vi "Build Blocks Tree.vi"(8 "error in (no error)":errorcluster, 10 "Blocks Map":map{string, T1}(c390), 11 "Blocks Tree":refnum<vi>) -> (0 "error out":errorcluster)   [LabVIEW 2022 SP3, in "FlexBlocks Support.lvlib"]
uses:
  FlexBlocks Support.lvlib
  Worker Info.ctl
  <vilib>/picture/picture.llb/imagedata.ctl
  Worker Variant.ctl
  <vilib>/Utility/miscctls.llb/LVMapReplaceAction.ctl
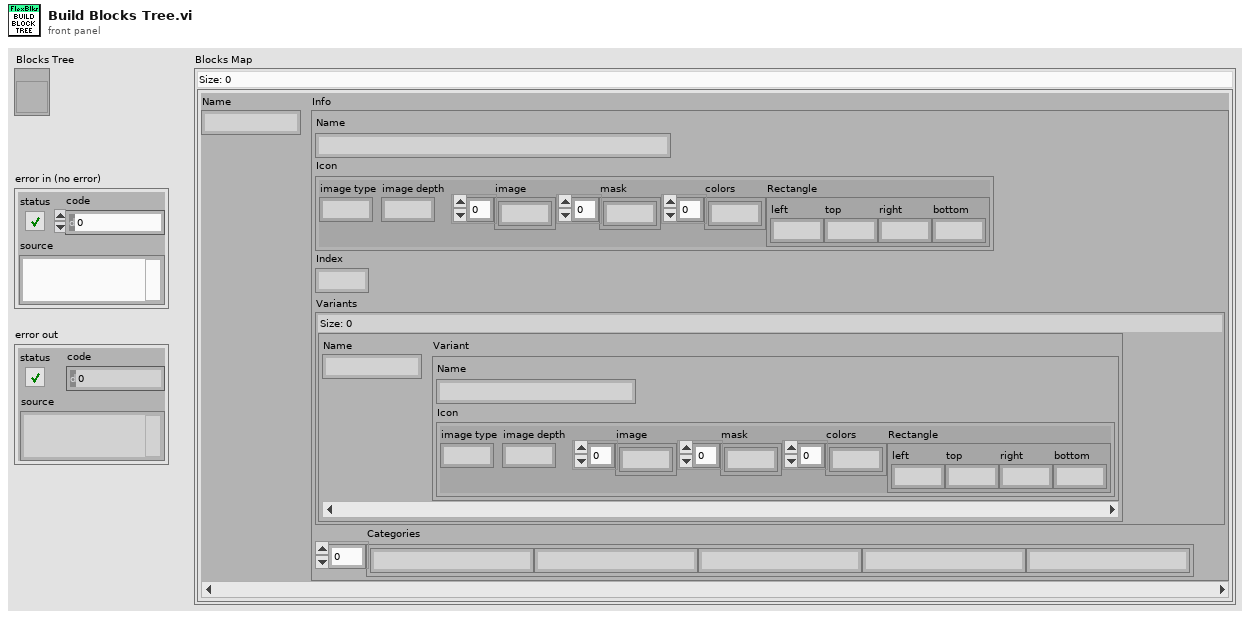
[diagram p1: front panel]
types:
  T1 = typedef "FlexBlocks Support.lvlib/Worker Info.ctl" = cluster{"Name":string, "Icon":T2, "Index":i32, "Variants":map{string, T3}, "Categories":string[]}
  T2 = typedef "imagedata.ctl" = cluster{"image type":i32, "image depth":i32, "image":u8[], "mask":u8[], "colors":u32[], "Rectangle":cluster{"left":i16, "top":i16, "right":i16, "bottom":i16}}
  T3 = typedef "FlexBlocks Support.lvlib/Worker Variant.ctl" = cluster{"Name":string, "Icon":T2}
  T4 = typedef "LVMapReplaceAction.ctl" = enum32{"Modify Entry only if found", "Add or Modify Entry", "Delete Entry"}
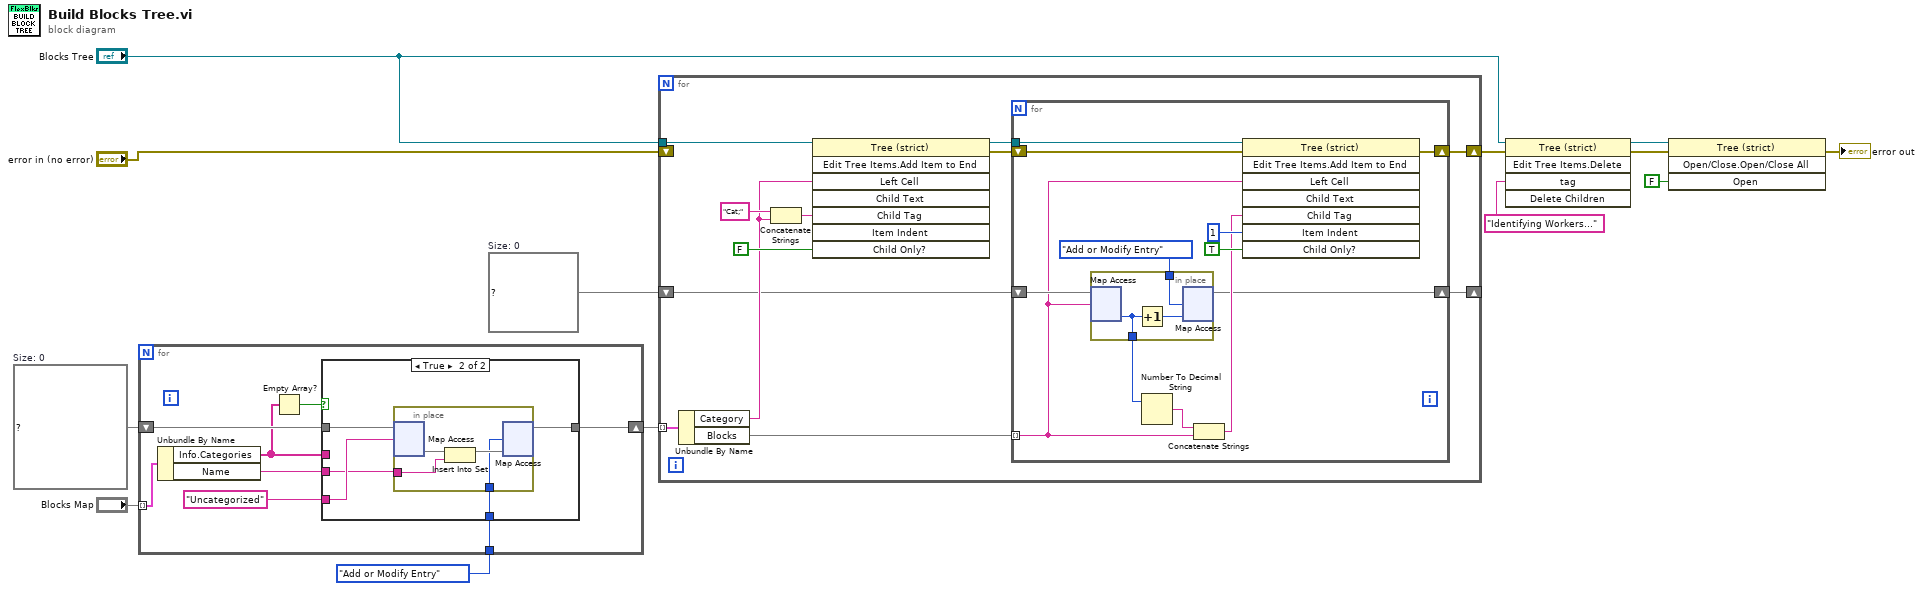
[diagram p0: block diagram]
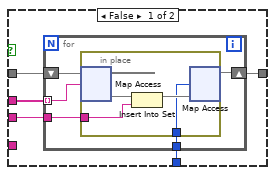
[diagram p2: hidden frame]
diagram:
  w9 = map{string, i32} {}  # Size: 0
  w12 = map{string, set{string}} {}  # Size: 0
  n1 = for {
    tunnel: "Blocks Map" -> [w21] mode=indexing
    shift-right: [w19] -> w10
    shift-left: w12 -> [w20]
    tunnel: LVMapReplaceAction."Add or Modify Entry" ("action") -> [w17]
    n2 = Unbundle By Name(w21) -> ("Info.Categories"=w16:string[], "Name"=w18:string)
    n3 = Empty Array?(array=w16) -> (empty?=w15:bool)
    n4 = case shown="True" w15 {
      tunnel: w20 -> [w26 w40]
      tunnel: [w25 w39] -> w19
      tunnel: w18 -> [w24 w36]
      tunnel: w17 -> [w23 w38]
      tunnel: w16 -> [w22 _]
      tunnel: "Uncategorized" -> [_ w37]
      frame False {
        n5 = for {
          shift-right: [w29] -> w25
          shift-left: w26 -> [w31]
          tunnel: w24 -> [w30]
          tunnel: w22 -> [w27] mode=indexing
          tunnel: w23 -> [w28]
          n6 = in-place {
            in-place-border: w30 -> [w34]
            in-place-border: w28 -> [w32]
            n7 = in-place-map #1(w31, w27) -> (w35:set{string})  [unwired: 1 in, 1 out]
            n8 = Insert Into Set(10:w34, 11:w35) -> (3:w33:set{string})  [unwired: 1 out]
            n9 = in-place-map #1(w33, w32) -> (w29:map{string, set{string}})  [unwired: 2 out]
          }
        }
      }
      frame True {
        n10 = in-place {
          in-place-border: w36 -> [w43]
          in-place-border: w38 -> [w41]
          n11 = in-place-map #2(w40, w37) -> (w44:set{string})  [unwired: 1 in, 1 out]
          n12 = Insert Into Set(10:w43, 11:w44) -> (3:w42:set{string})  [unwired: 1 out]
          n13 = in-place-map #2(w42, w41) -> (w39:map{string, set{string}})  [unwired: 2 out]
        }
      }
    }
  }
  n14 = for {
    tunnel: w10 -> [w56] mode=indexing
    shift-right: [w45] -> _
    shift-left: w9 -> [w47]
    tunnel: "Blocks Tree" -> [w55]
    shift-right: [w48] -> w6
    shift-left: "error in (no error)" -> [_]
    n15 = Unbundle By Name(w56) -> ("Category"=w51:string, "Blocks"=w46:set{string})
    n16 = Concatenate Strings("Cat;" ("string"), w51) -> (w53:string)
    n17 = invoke class="Tree (strict)" method="Edit Tree Items.Add Item to End"(reference=w55, "Left Cell"=w51, "Child Tag"=w53, "Child Only?"=FALSE) -> (reference out=w50:refnum<vi>, error out=w49:errorcluster)  [unwired: 4 in, 6 out]
    n18 = for {
      tunnel: w50 -> [w67]
      shift-right: [w57] -> w48
      shift-left: w49 -> [w68]
      shift-right: [w58] -> w45
      shift-left: w47 -> [w64]
      tunnel: w46 -> [w61] mode=indexing
      n19 = in-place {
        in-place-border: LVMapReplaceAction."Add or Modify Entry" ("action") -> [w71]
        in-place-border: [w69] -> w62
        n20 = in-place-map #3(w64, w61) -> (w69:i32)  [unwired: 1 in, 1 out]
        n21 = Increment(x=w69) -> (x+1=w70:i32)
        n22 = in-place-map #3(w70, w71) -> (w58:map{string, i32})  [unwired: 2 out]
      }
      n23 = Number To Decimal String(number=w62) -> (decimal integer string=w60:string)  [unwired: 1 in]
      n24 = Concatenate Strings(w60, w61) -> (w59:string)
      n25 = invoke class="Tree (strict)" method="Edit Tree Items.Add Item to End"(reference=w67, error in=w68, "Left Cell"=w61, "Child Tag"=w59, "Item Indent"=1 ("New Item Indentation"), "Child Only?"=TRUE) -> (error out=w57:errorcluster)  [unwired: 2 in, 7 out]
    }
  }
  n26 = invoke class="Tree (strict)" method="Edit Tree Items.Delete"(reference="Blocks Tree", error in=w6, "tag"="Identifying Workers...") -> (reference out=w4:refnum<vi>, error out=w2:errorcluster)  [unwired: 2 in, 3 out]
  n27 = invoke class="Tree (strict)" method="Open/Close.Open/Close All"(reference=w4, error in=w2, "Open"=FALSE ("Open?")) -> (error out=→"error out":errorcluster)  [unwired: 1 in, 3 out]
